vi "Packetize.vi"(8 "Error In":errorcluster, 10 "Data":u8[](array[numeric]), 11 "Arduino Resource":T1={"COM Port"="", "Board Type"=enum."ChipKit Uno32", "Connection Type"=enum."USB / Serial", "Baud Rate (115200)"=15, "Bytes Per Packet (15)"=15, "DI Port Num Pins"=0, "DO Port Num Pins"=0}) -> (0 "Error Out":errorcluster, 2 "Packet":string, 3 "Arduino Resource":T1={"COM Port"="", "Board Type"=enum."ChipKit Uno32", "Connection Type"=enum."USB / Serial", "Baud Rate (115200)"=15, "Bytes Per Packet (15)"=15, "DI Port Num Pins"=0, "DO Port Num Pins"=0})   [LabVIEW 2011, in "LabVIEW Interface for ChipKit.lvlib"]
doc: "Pack data into packets including checksum and ensure fixed packet length."
uses:
  LabVIEW Interface for ChipKit.lvlib
  Private/Type Defs/Chipkit Resource.ctl
  Private/Type Defs/Board Type.ctl
  Private/Type Defs/Connection Type.ctl
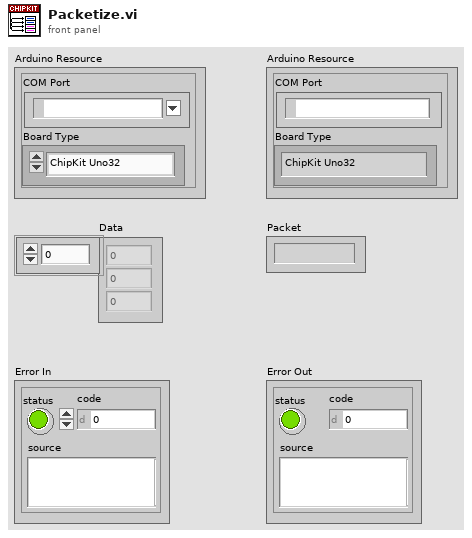
[diagram p1: front panel]
types:
  T1 = typedef "LabVIEW Interface for ChipKit.lvlib/Chipkit Resource.ctl" = cluster{"COM Port":refnum<visa-resource-name>, "Board Type":T2, "Connection Type":T3, "Baud Rate (115200)":u32, "Bytes Per Packet (15)":u32, "DI Port Num Pins":i32, "DO Port Num Pins":i32}
  T2 = typedef "LabVIEW Interface for ChipKit.lvlib/Board Type.ctl" = enum16{"ChipKit uC32", "ChipKit Uno32", "ChipKit Max32"}
  T3 = typedef "LabVIEW Interface for ChipKit.lvlib/Connection Type.ctl" = enum8{"USB / Serial", "XBEE", "BlueSmirf (Bluetooth)"}
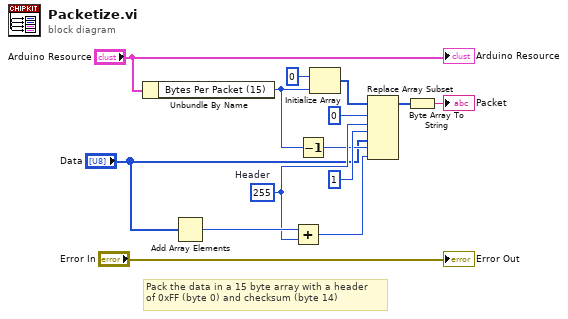
[diagram p0: block diagram]
diagram:
  w8 = u8 255  # Header
  # "Pack the data in a 15 byte array with a header \nof 0xFF (byte 0) and checksum (byte 14)"
  n1 = Unbundle By Name("Arduino Resource") -> ("Bytes Per Packet (15)"=w4:u32)
  n2 = Add Array Elements(numeric array="Data") -> (sum=w9:u8)
  n3 = Add(x=w9, y=w8) -> (x+y=w7:u8)
  n4 = Decrement(x=w4) -> (x-1=w5:u32)
  n5 = Initialize Array(u8 0, w4) -> (w14:u8[])
  n6 = Replace Array Subset(array=w14, new element #1=w8, index #1=0 ("index"), new element #2="Data", index #2=1 ("index"), new element #3=w7, index #3=w5) -> (w6:u8[])
  n7 = Byte Array To String(unsigned byte array=w6) -> (string=→"Packet":string)
  "Arduino Resource" <- "Arduino Resource"
  "Error Out" <- "Error In"
